vi "Query Active DUT Band Restrictions Catalog.vi"(8 "error in (no error)":errorcluster, 11 "VISA resource name":refnum<visa-resource-name>) -> (0 "error out":errorcluster, 2 "Band Restrictions":string, 3 "VISA resource name out":refnum<visa-resource-name>)   [LabVIEW 2015, in "Rohde&Schwarz CMXP Base.lvlib"]
doc: "Queries the DUT connector restrictions for the active DUT.\n\nAttribute:\nRSCMXPBASE_ATTR_ACTIVE_DUT_BAND_RESTRICTIONS_CATALOG\n\nRemote-control command:\nCATalog:DUT:BAND:RESTrictions?"
uses:
  <instrlib>/Rohde&Schwarz CMXP Base/Rohde&Schwarz CMXP Base.lvlib
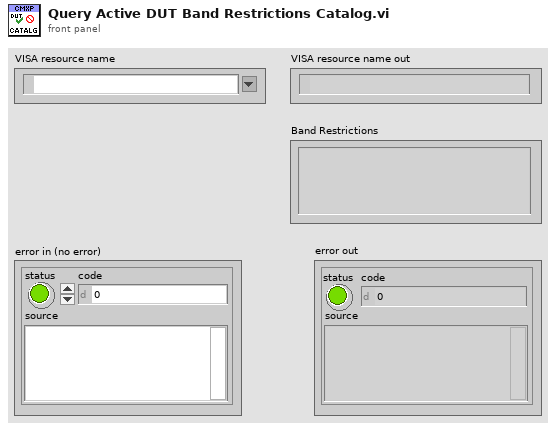
[diagram p1: front panel]
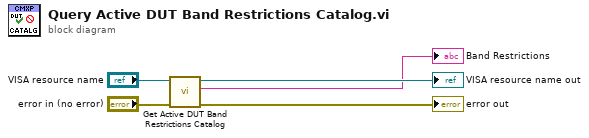
[diagram p0: block diagram]
diagram:
  n1 = call "Get Active DUT Band Restrictions Catalog"("error in (no error)"="error in (no error)", "instrument handle"="VISA resource name") -> ("error out"=→"error out":errorcluster, "Active DUT Band Restrictions Catalog"=→"Band Restrictions":string, "instrument handle out"=→"VISA resource name out":refnum<visa-resource-name>)  [unwired: 7 in]
